vi "HMI CSE1.vi"() -> ()   [LabVIEW 2010]
uses:
  <vilib>/addons/Simulation Interface/_sitctls/sit Indicator Info.ctl
  <vilib>/addons/Simulation Interface/_sitctls/sit Indicator Type.ctl
  <vilib>/addons/Simulation Interface/_sitctls/sit Client Meta Info (v3).ctl
  <vilib>/addons/Simulation Interface/_sitctls/sit MDL Line Item Info.ctl
  <vilib>/addons/Simulation Interface/_sitctls/sit MDL Line Type.ctl
  <vilib>/addons/Simulation Interface/_sitctls/sit Details Settings.ctl
  <vilib>/addons/Simulation Interface/_sitctls/sit Execution Host.ctl
  <vilib>/addons/Simulation Interface/_sitctls/SIT Sim State.ctl
  <vilib>/Utility/inputDevices.llb/closeJoystick.vi
  <vilib>/Utility/inputDevices.llb/joystickAcquire.vi
  <vilib>/addons/Simulation Interface/_sitclient.llb/NI_SIT_sitclient.lvlib
  <vilib>/addons/Simulation Interface/_sitctls/NI_SIT_sitctls.lvlib
  <vilib>/ptbypt/NI_PtbyPt.lvlib
  <vilib>/picture/3D Picture Control/NI_3D Picture Control.lvlib
panel:
  out "Navigation eta yaw":dbl
  out "Navigation eta sway":dbl
  out "Navigation eta surge":dbl
  out "Plant u5":dbl
  out "Plant u4":dbl
  out "Plant u3":dbl
  out "Plant u2":dbl
  out "Plant u1":dbl
  out "DP eta Psi deg":dbl
  out "DP eta E":dbl
  out "DP eta N":dbl
  out "DP eta_d Psi deg":dbl
  out "DP eta_d E":dbl
  out "DP eta_d N":dbl
  in  "Enabler":bool
  in  "Enable Linear Simulator":bool
  in  "Control Input Selector":enum32{"OK Button 4", "OK Button 5"}(radio)
  in  "MODE":T1(radio)=enum."OK Button 4"
  in  "Enable CSE1 actuator":bool
  in  "SIT_RVE":bool
  in  "SIT_Remap":bool
  in  "SIT_Details":bool
  in  "SIT_Stop":bool
  in  "SIT_Pause":bool
  in  "SIT_Run":bool
  in  "SIT_stopVI":bool
  out "SIT_Status":string
  in  "Tab Front Pannel":T2(tab)
  in  "u5":dbl
  in  "u4":dbl
  in  "u3":dbl
  in  "u2":dbl
  in  "u1":dbl
  in  "VSP Speed":dbl(slide) min=-1.0 max=1.0 step=0.05 scale=-1.0..1.0 scale format="%#_2g"
  in  "BT Power Limiter":dbl(slide) min=0.0 max=1.0 step=0.1 scale=-1.0..1.0
  in  "Left Y":dbl(slide) scale=-35860.0..35860.0
  in  "Left X":dbl(slide) scale=-35860.0..35860.0
  in  "Right X":dbl(slide) scale=-35860.0..35860.0
  in  "Right Y":dbl(slide) scale=-35860.0..35860.0
  out "Servo Battery":dbl(knob) scale=0.0..8.0
  out "Bowthruster Battery":dbl(knob) scale=0.0..8.0
  out "Main Battery":dbl(knob) scale=0.0..18.0
  out "Left Joystick":bool
  out "Right Joystick":bool
  out "Direction Up":bool
  out "Direction Right":bool
  out "Direction Down":bool
  out "Direction Left":bool
  out "L2 Button":bool
  out "R2 Button":bool
  out "Triangle Button":bool
  out "Circle Button":bool
  out "X Button":bool
  out "Square Button":bool
  out "Joystick Info":T3(array[cluster])
  in  "L2":sgl
  in  "R2":sgl
  out "Slide BT red":dbl(slide)
  out "Slide BT green":dbl(slide) scale=0.0..1.0
  out "Magnitude Pitch Starboard VSP":dbl(knob) scale=0.0..1.0
  out "Magnitude Pitch Port VSP":dbl(knob) scale=0.0..1.0
  out "Direction Starboard VSP":dbl(knob) scale=180.0..-180.0
  out "Direction Port VSP":dbl(knob) scale=180.0..-180.0
  in  "Acccuracy BT":dbl
  in  "Accuracy VSP":dbl
  in  "Tab Plants":enum32{"eta", "Qualisys", "Linear Simulator"}(tab)
  in  "Tab eta":enum32{"Navigation output", "Qualisys"}(tab)
  out "Iceberg yaw":dbl
  out "Iceberg pitch":dbl
  out "Iceberg roll":dbl
  out "Iceberg z-position":dbl
  out "Iceberg y-position":dbl
  out "Iceberg x-position":dbl
  out "CSE1 yaw [rad]":dbl
  out "CSE1 pitch [rad]":dbl
  out "CSE1 roll [rad]":dbl
  out "CSE1 z-position [m]":dbl
  out "CSE1 y-position [m]":dbl
  out "CSE1 x-position [m]":dbl
  out "QS yaw [rad]":dbl
  out "QS pitch [rad]":dbl
  out "QS roll [rad]":dbl
  out "QS z-position [m]":dbl
  out "QS y-position [m]":dbl
  out "QS x-position [m]":dbl
  in  "Show CSEI":bool
  in  "Show Iceberg":bool
  out "QTM In9":dbl
  out "QTM In8":dbl
  out "QTM In7":dbl
  out "QTM In6":dbl
  out "QTM In5":dbl
  out "QTM In4":dbl
  out "QTM In3":dbl
  out "QTM In2":dbl
  out "QTM In1":dbl
  out "LS nu_yaw_hil":dbl
  out "LS nu_sway_hil":dbl
  out "LS nu_surge_hil":dbl
  out "LS etadot_yaw_hil":dbl
  out "LS etadot_sway_hil":dbl
  out "LS etadot_surge_hil":dbl
  out "LS eta_yaw_hil":dbl
  out "LS eta_sway_hil":dbl
  out "LS  eta_surge_hil":dbl
  in  "LS r_0":dbl
  in  "LS v_0":dbl
  in  "LS u_0":dbl
  in  "LS psi_0":dbl
  in  "LS y_0":dbl
  in  "LS x_0":dbl
  in  "Button Reset HIL Integrator":bool
  in  "Reset Linear Simulator integrator":dbl
  in  "Tab Control system":enum32{"DP Control", "Page 2"}(tab)
  in  "DP Wave Filter":bool
  in  "DP eta_d LPF":bool
  in  "DP K_d Scale":dbl(slide) min=0.0 max=5.0 step=0.25 scale=0.0..5.0
  in  "DP K_i Scale":dbl(slide) min=0.0 max=5.0 step=0.25 scale=0.0..5.0
  in  "DP K_p Scale":dbl(slide) min=0.0 max=10.0 step=0.5 scale=0.0..10.0
  in  "DP eta_d_N [m]":dbl
  in  "DP eta_d_E [m]":dbl
  in  "Button Reset DP Integrator.":bool
  in  "DP eta_d_Psi [deg]":dbl(knob) scale=0.0..360.0 scale format="%#.3p"
  out "Ind eta_d_Psi [rad]":dbl format="%#_2g"
  in  "Reset DP Integrator":dbl
  out "3D Picture":refnum<vi>(3d-picture)
  in  "Tab Reg plots":enum32{"DP", "Page 2"}(tab)
  out "DP Reponse N":cluster{"Value":dbl, "Value":dbl}(graph)
  out "DP Error N":waveform(dbl)[](graph)
  out "DP Error E":waveform(dbl)[](graph)
  out "DP Error Psi":waveform(dbl)[](graph)
  out "DP Reponse Psi":cluster{"Value":dbl, "Value":dbl}(graph)
  out "DP Response E":cluster{"Value":dbl, "Value":dbl}(graph)
  in  "Tab Command":enum32{"DP", "Page 2"}(tab)
  out "DP tau surge":waveform(dbl)[](graph)
  out "DP tau sway":waveform(dbl)[](graph)
  out "DP tau yaw":waveform(dbl)[](graph)
  out "DP u_1":waveform(dbl)[](graph)
  out "DP u_2":waveform(dbl)[](graph)
  out "DP u_3":waveform(dbl)[](graph)
  out "DP u_4":waveform(dbl)[](graph)
  out "DP u_5":waveform(dbl)[](graph)
  in  "SIT_Meta_Info":T4
  in  "SIT_Indicator_Indices":T9[](array[typedef])=[{"Indicator Index"=0, "Number of Signals"=1, "Indicator Type"=enum."Knob"}, {"Indicator Index"=-1, "Number of Signals"=0, "Indicator Type"=enum."Digital"}, {"Indicator Index"=-1, "Number of Signals"=0, "Indicator Type"=enum."Digital"}, {"Indicator Index"=3, "Number of Signals"=1, "Indicator Type"=enum."Digital"}, {"Indicator Index"=4, "Number of Signals"=1, "Indicator Type"=enum."Digital"}, {"Indicator Index"=5, "Number of Signals"=1, "Indicator Type"=enum."Digital"}, {"Indicator Index"=-1, "Number of Signals"=0, "Indicator Type"=enum."Digital"}, {"Indicator Index"=7, "Number of Signals"=1, "Indicator Type"=enum."WaveformChart"}, {"Indicator Index"=8, "Number of Signals"=1, "Indicator Type"=enum."WaveformChart"}, {"Indicator Index"=9, "Number of Signals"=1, "Indicator Type"=enum."WaveformChart"}, {"Indicator Index"=10, "Number of Signals"=1, "Indicator Type"=enum."Digital"}, {"Indicator Index"=11, "Number of Signals"=1, "Indicator Type"=enum."Digital"}, {"Indicator Index"=12, "Number of Signals"=1, "Indicator Type"=enum."Digital"}, {"Indicator Index"=13, "Number of Signals"=1, "Indicator Type"=enum."Digital"}, {"Indicator Index"=14, "Number of Signals"=1, "Indicator Type"=enum."Digital"}, {"Indicator Index"=15, "Number of Signals"=1, "Indicator Type"=enum."Digital"}, {"Indicator Index"=16, "Number of Signals"=1, "Indicator Type"=enum."WaveformChart"}, {"Indicator Index"=17, "Number of Signals"=1, "Indicator Type"=enum."WaveformChart"}, {"Indicator Index"=18, "Number of Signals"=1, "Indicator Type"=enum."WaveformChart"}, {"Indicator Index"=19, "Number of Signals"=1, "Indicator Type"=enum."WaveformChart"}, {"Indicator Index"=20, "Number of Signals"=1, "Indicator Type"=enum."WaveformChart"}, {"Indicator Index"=21, "Number of Signals"=1, "Indicator Type"=enum."WaveformChart"}, {"Indicator Index"=22, "Number of Signals"=1, "Indicator Type"=enum."WaveformChart"}, {"Indicator Index"=23, "Number of Signals"=1, "Indicator Type"=enum."WaveformChart"}, {"Indicator Index"=24, "Number of Signals"=1, "Indicator Type"=enum."Knob"}, {"Indicator Index"=25, "Number of Signals"=1, "Indicator Type"=enum."Knob"}, {"Indicator Index"=-1, "Number of Signals"=0, "Indicator Type"=enum."Digital"}, {"Indicator Index"=-1, "Number of Signals"=0, "Indicator Type"=enum."Digital"}, {"Indicator Index"=-1, "Number of Signals"=0, "Indicator Type"=enum."Digital"}, {"Indicator Index"=-1, "Number of Signals"=0, "Indicator Type"=enum."Digital"}, {"Indicator Index"=-1, "Number of Signals"=0, "Indicator Type"=enum."Digital"}, {"Indicator Index"=-1, "Number of Signals"=0, "Indicator Type"=enum."Digital"}, {"Indicator Index"=32, "Number of Signals"=1, "Indicator Type"=enum."Digital"}, {"Indicator Index"=33, "Number of Signals"=1, "Indicator Type"=enum."Digital"}, {"Indicator Index"=34, "Number of Signals"=1, "Indicator Type"=enum."Digital"}, {"Indicator Index"=35, "Number of Signals"=1, "Indicator Type"=enum."Digital"}, {"Indicator Index"=36, "Number of Signals"=1, "Indicator Type"=enum."Digital"}, {"Indicator Index"=37, "Number of Signals"=1, "Indicator Type"=enum."Digital"}, {"Indicator Index"=38, "Number of Signals"=1, "Indicator Type"=enum."Digital"}, {"Indicator Index"=39, "Number of Signals"=1, "Indicator Type"=enum."Digital"}, {"Indicator Index"=40, "Number of Signals"=1, "Indicator Type"=enum."Digital"}, {"Indicator Index"=41, "Number of Signals"=1, "Indicator Type"=enum."Knob"}, {"Indicator Index"=42, "Number of Signals"=1, "Indicator Type"=enum."Knob"}, {"Indicator Index"=43, "Number of Signals"=1, "Indicator Type"=enum."Knob"}, {"Indicator Index"=44, "Number of Signals"=1, "Indicator Type"=enum."Digital"}, {"Indicator Index"=45, "Number of Signals"=1, "Indicator Type"=enum."Digital"}, {"Indicator Index"=46, "Number of Signals"=1, "Indicator Type"=enum."Digital"}, {"Indicator Index"=47, "Number of Signals"=1, "Indicator Type"=enum."Digital"}, {"Indicator Index"=48, "Number of Signals"=1, "Indicator Type"=enum."Digital"}, {"Indicator Index"=49, "Number of Signals"=1, "Indicator Type"=enum."Digital"}, {"Indicator Index"=50, "Number of Signals"=1, "Indicator Type"=enum."Digital"}, {"Indicator Index"=51, "Number of Signals"=1, "Indicator Type"=enum."Digital"}, {"Indicator Index"=52, "Number of Signals"=1, "Indicator Type"=enum."Digital"}, {"Indicator Index"=53, "Number of Signals"=1, "Indicator Type"=enum."Digital"}, {"Indicator Index"=54, "Number of Signals"=1, "Indicator Type"=enum."Digital"}, {"Indicator Index"=55, "Number of Signals"=1, "Indicator Type"=enum."Digital"}, {"Indicator Index"=56, "Number of Signals"=1, "Indicator Type"=enum."Digital"}, {"Indicator Index"=57, "Number of Signals"=1, "Indicator Type"=enum."Digital"}, {"Indicator Index"=58, "Number of Signals"=1, "Indicator Type"=enum."Digital"}, {"Indicator Index"=59, "Number of Signals"=1, "Indicator Type"=enum."Digital"}, {"Indicator Index"=60, "Number of Signals"=1, "Indicator Type"=enum."Digital"}, {"Indicator Index"=61, "Number of Signals"=1, "Indicator Type"=enum."Digital"}, {"Indicator Index"=62, "Number of Signals"=1, "Indicator Type"=enum."Digital"}, {"Indicator Index"=63, "Number of Signals"=1, "Indicator Type"=enum."Digital"}, {"Indicator Index"=64, "Number of Signals"=1, "Indicator Type"=enum."Digital"}, {"Indicator Index"=65, "Number of Signals"=1, "Indicator Type"=enum."Digital"}, {"Indicator Index"=66, "Number of Signals"=1, "Indicator Type"=enum."Digital"}, {"Indicator Index"=67, "Number of Signals"=1, "Indicator Type"=enum."Knob"}, {"Indicator Index"=68, "Number of Signals"=1, "Indicator Type"=enum."Slide"}, {"Indicator Index"=69, "Number of Signals"=1, "Indicator Type"=enum."Slide"}]
  # "MODE"
  # "Controller Input Selector"
  # "TARGET"
  # "Model Controls"
  # "VSP Speed"
  # "VSP speed = 1\n\nStarboard VSP\nMax Speed  ClockWise\n\nPort VSP \nMax Speed CounterClockWise"
  # "VSP Speed = -1\n\nStarboard VSP \nMax Speed CounterClockWise\n\nPort VSP\nMax Speed ClockWise"
  # "Bow Thruster Power Limit"
  # "Max Power"
  # "Max Power"
  # "No Power"
  # "PS3 Joysticks"
  # "Increase BT power limit"
  # "Increase VSP speed"
  # "Decrease BT power limit"
  # "Decrease VSP speed"
  # "Port VSP\n(surge/sway force setpoint)"
  # "Starboard VSP"
  # "Bowthruster"
  # "VSP pitch"
  # "CS Enterprise I"
  # "Toggle visibility"
  # "Iceberg"
  # "Toggle visibility"
  # "Initial eta"
  # "Initial nu"
  # "DP controller gains"
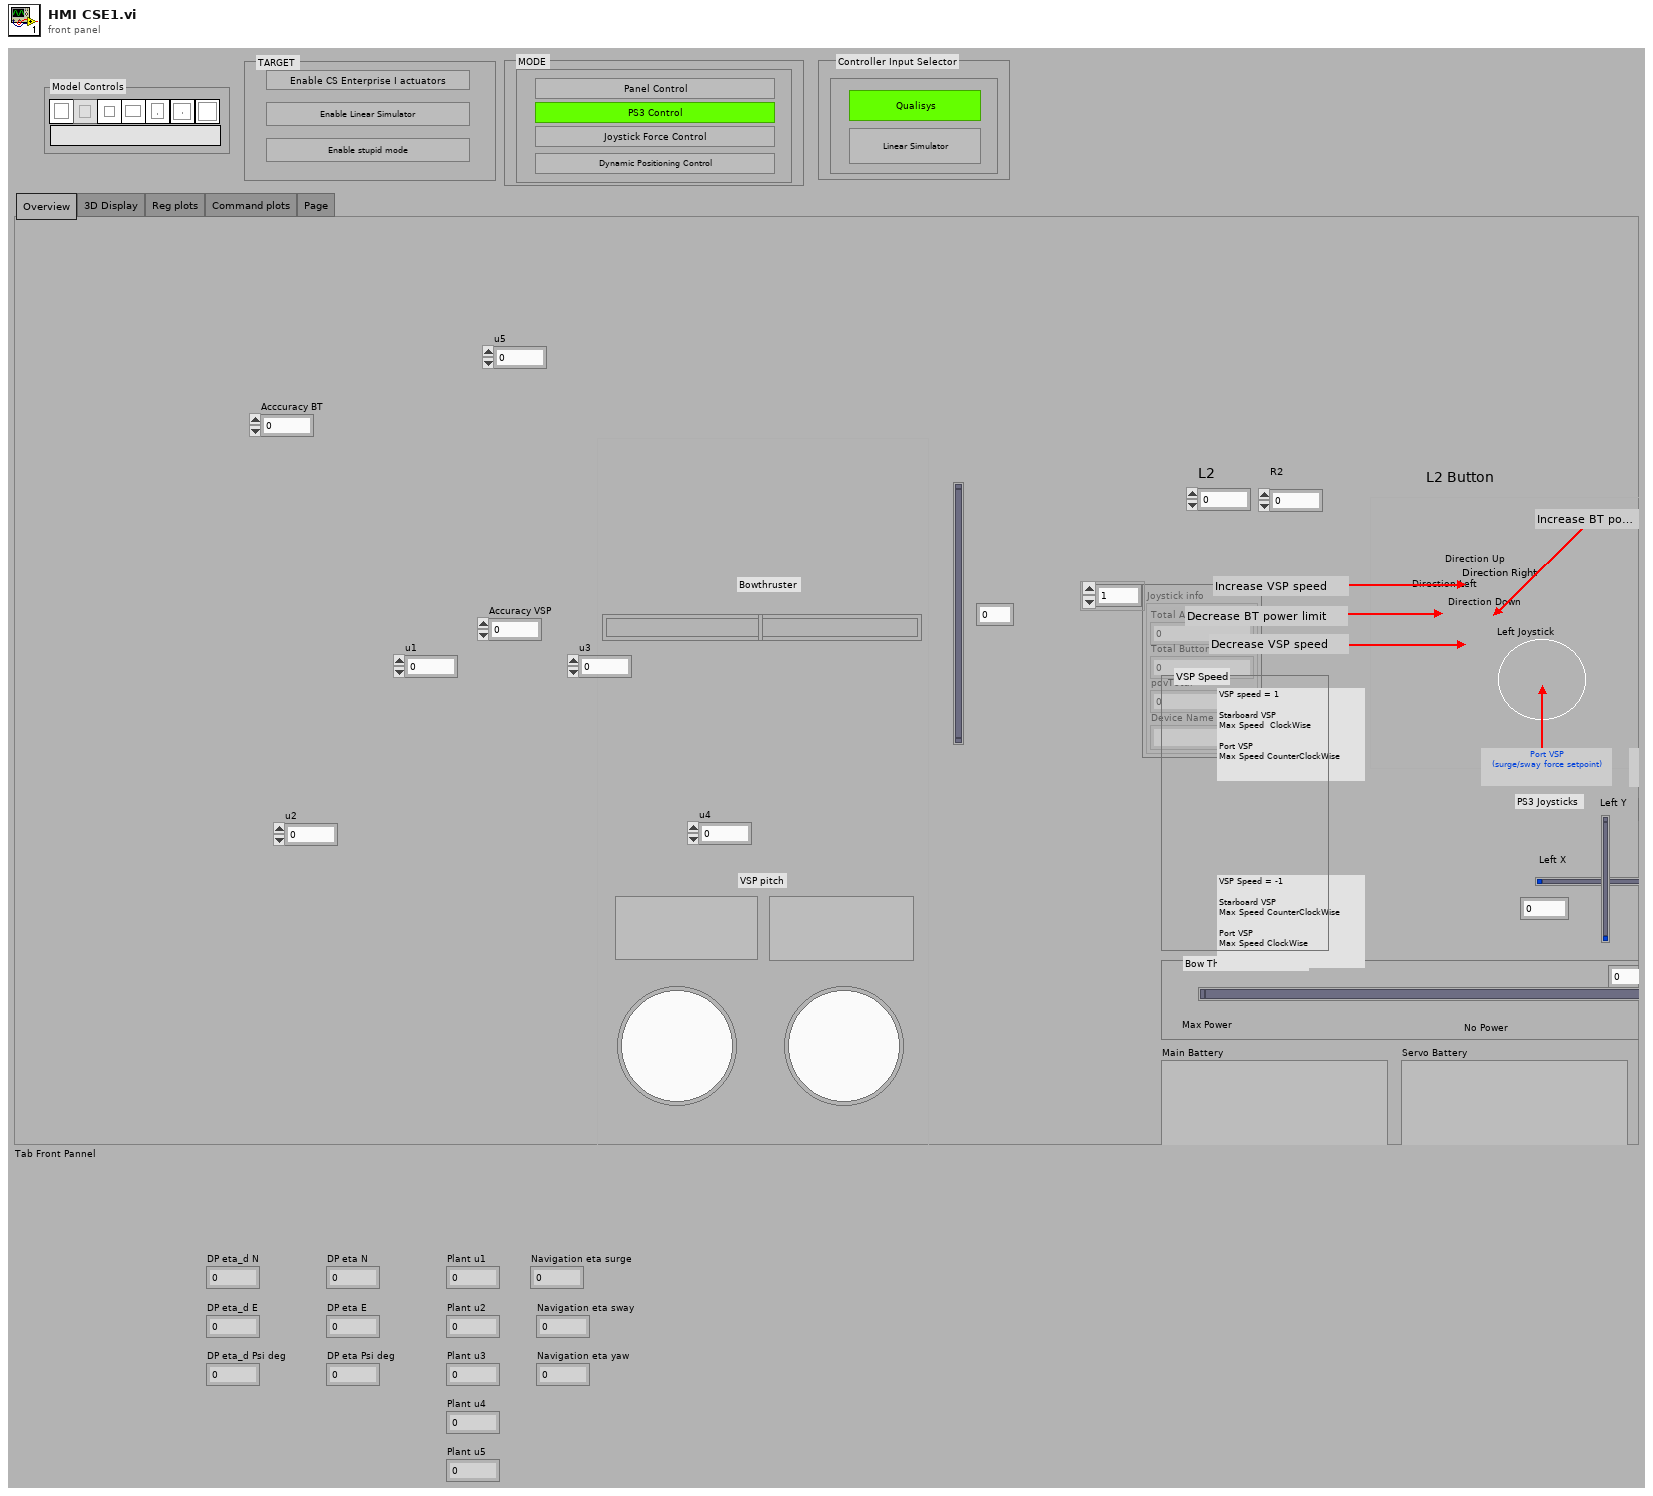
[diagram p1: front panel]
types:
  T1 = enum32{"Radio Selection 4", "OK Button 4", "OK Button 5", "OK Button 6"}
  T2 = enum32{"Overview", "3D Display", "Reg plots", "Command plots", "Page"}
  T3 = cluster{"Total Axis":u32, "Total Buttons":u32, "povTotal":u32, "Device Name":string}[]
  T4 = typedef "NI_SIT_sitctls.lvlib/sit Client Meta Info (v3).ctl" = cluster{"Simulation IP":string, "Target IP":string, "Host Port":u16, "Model DLL Path":path, "Model File Path":path, "Model Name":string, "Param Tree Info ":T5[], "Signal Tree Info":T5[], "Details Settings":T7, "Client Name":string, "Stored Model Checksum":string, "Buffer Sizes":cluster{"number of signals":u32, "circular buffer size":u32, "num data points":u32}, "Execution Host":T8, "Project Dir":path, "Last MDL":path}
  T5 = typedef "NI_SIT_sitctls.lvlib/sit MDL Line Item Info.ctl" = cluster{"Line Type":T6, "Section Type":string, "Name":string, "Value":string, "Owner Index":i32, "Tree Tag":string, "Child Indices":i32[], "Expanded?":bool, "Destination Block Info":string[]}
  T6 = typedef "NI_SIT_sitctls.lvlib/sit MDL Line Type.ctl" = enum16{"Section Head", "Parameter", "Section End", "Comment"}
  T7 = typedef "NI_SIT_sitctls.lvlib/sit Details Settings.ctl" = cluster{"Halt on Task Overrun?":bool, "Halt on Lost Data?":bool, "Signal Decimation":i32, "Autoscale":bool}
  T8 = typedef "NI_SIT_sitctls.lvlib/sit Execution Host.ctl" = enum32{"Simulation Environment", "RT Target", "Local Driver"}
  T9 = typedef "NI_SIT_sitctls.lvlib/sit Indicator Info.ctl" = cluster{"Indicator Index":i32, "Number of Signals":i32, "Indicator Type":T10}
  T10 = typedef "NI_SIT_sitctls.lvlib/sit Indicator Type.ctl" = enum32{"xxx1", "xxx2", "xxx3", "Generic   ", "Decoration", "Text", "xControl", "ColorBox", "Boolean", "RefNum", "Variant", "Path", "ListBox", "Table", "Array", "Picture", "ActiveXContainer", "Numeric", "Digital", "NamedNumeric", "ColorRamp", "Slide", "GraphOrChart", "WaveformChart", "WaveformGraph", "IntensityChart", "xxx4", "xxx5", "xxx6", "xxx7", "Cluster", "Panel", "Knob", "NumWithScale", "Ring", "Enum", "GObject", "Plot", "Cursor", "NumericText", "Scale", "ColorScale", "GraphScale", "ColorGraphScale", "TypedRefNum", "OldKnobScale", "MCListbox", "WaveformData", "BVTag", "DAQName", "VISAName", "IVIName", "SlideScale"}
  T11 = cluster{"Red":sgl, "Green":sgl, "Blue":sgl, "Alpha":sgl}
  T12 = cluster{"axes total":u32, "buttons total":u32, "pov total":u32, "device name":string}[]
  T13 = typedef "NI_SIT_sitctls.lvlib/sit TCP Conn and Queue.ctl" = cluster{"TCP Connection":refnum<k5>, "Data Queue":refnum<queue>, "Execution Host":T8}
  T14 = typedef "NI_SIT_sitctls.lvlib/sit Client Op Refs.ctl" = cluster{"Conn and Queue":T13, "RunPauseStop Refs":refnum<vi>[], "Control Refs":refnum<vi>[], "Indicator Refs":refnum<vi>[], "Param Info":T15[], "State Queue":refnum<queue>, "Don't Modify Scales?":bool, "Param Info Needs Init?":bool}
  T15 = typedef "NI_SIT_sitctls.lvlib/SIT param info.ctl" = cluster{"paramidx":i32, "ID":string, "paramname":string, "dattype":i32, "Dimensions":i32[], "value":dbl[]}
  T16 = typedef "NI_SIT_sitctls.lvlib/SIT Sim State.ctl" = enum8{"Default", "Idle", "Running", "Paused", "Stopped", "Error"}
  T17 = cluster{"X axis":i32, "Y axis":i32, "Z axis":i32, "X axis rotation":i32, "Y axis rotation":i32, "Z axis rotation":i32, "U axis":i32, "V axis":i32}
  T18 = cluster{"button 1":bool, "button 2":bool, "button 3":bool, "button 4":bool, "button 5":bool, "button 6":bool, "button 7":bool, "button 8":bool, "button 9":bool, "button 10":bool, "button 11":bool, "button 12":bool, "button 13":bool, "button 14":bool, "button 15":bool, "button 16":bool, "button 17":bool, "button 18":bool, "button 19":bool, "button 20":bool, "button 21":bool, "button 22":bool, "button 23":bool, "button 24":bool, "button 25":bool, "button 26":bool, "button 27":bool, "button 28":bool, "button 29":bool, "button 30":bool, "button 31":bool, "button 32":bool}
  T19 = cluster{"pov 1":i32, "pov 2":i32, "pov 3":i32, "pov 4":i32}
  T20 = cluster{"DP eta_d_N [m]":dbl, "Red":sgl, "DP eta_d_E [m]":dbl}
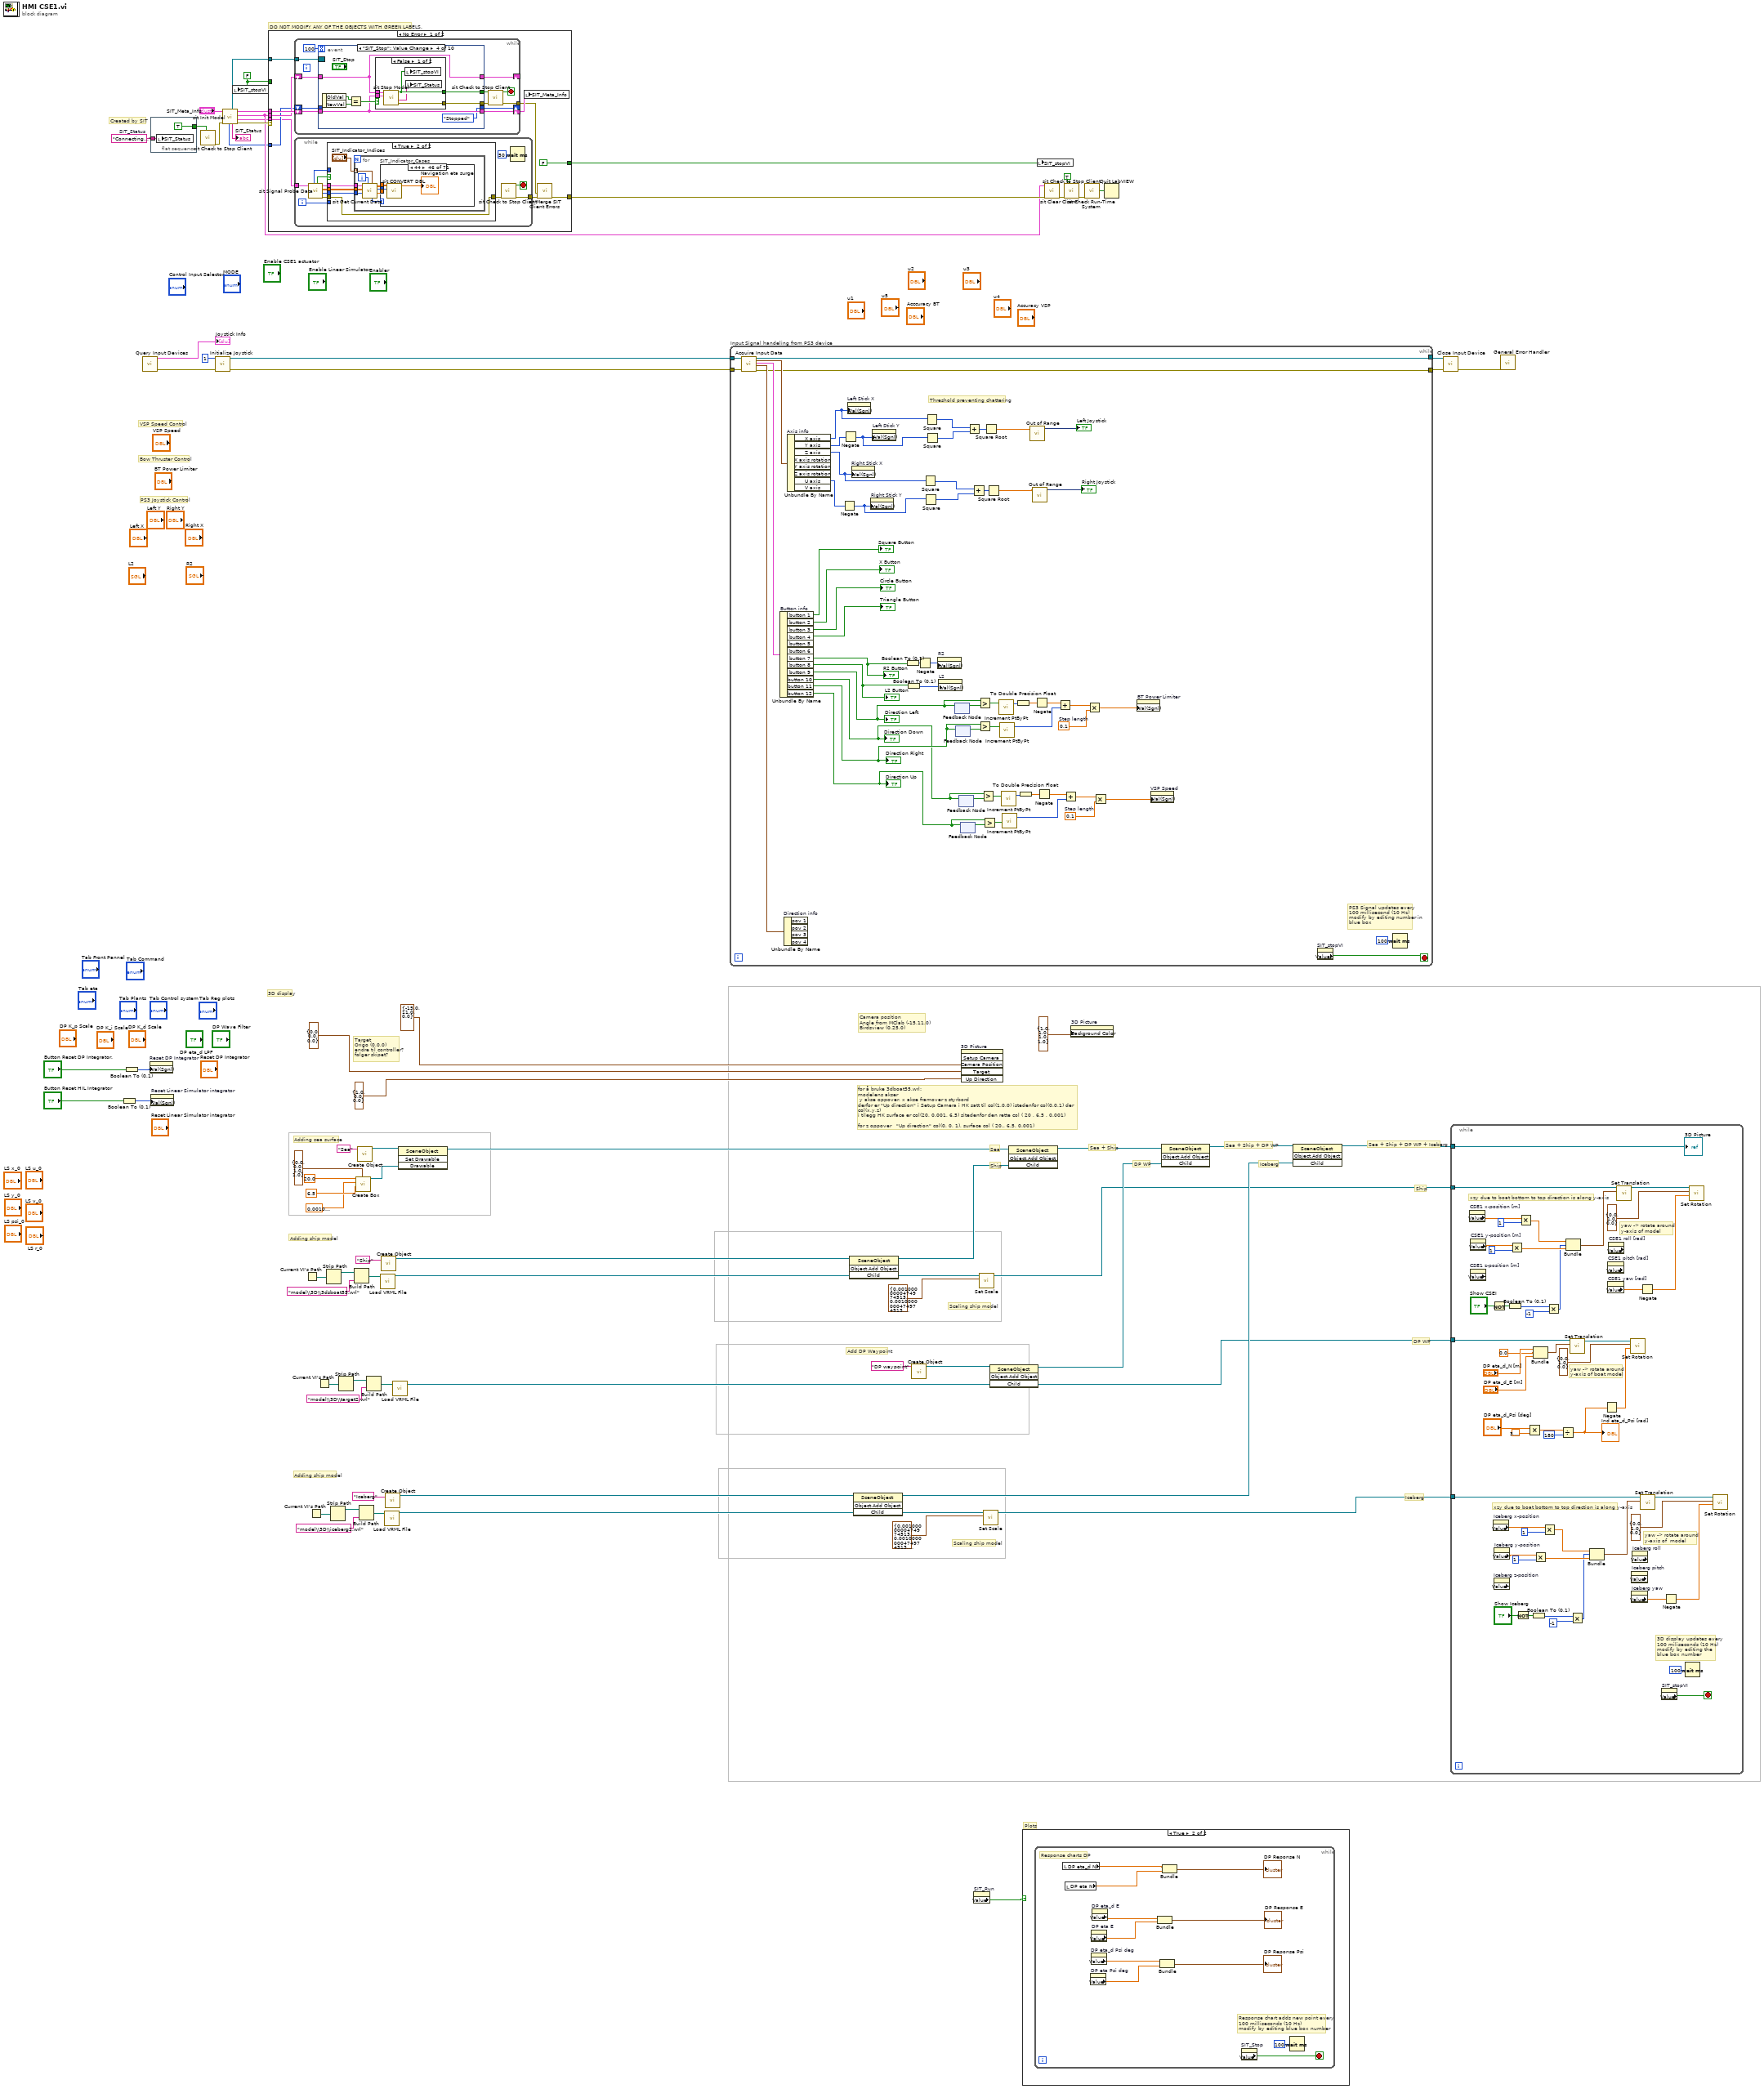
[diagram p0: block diagram]
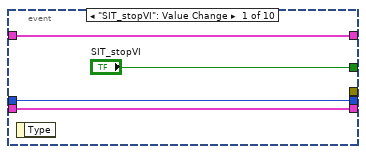
[diagram p3: hidden frame]
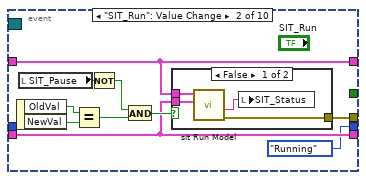
[diagram p4: hidden frame]
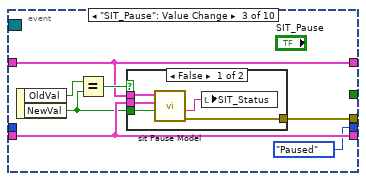
[diagram p6: hidden frame]
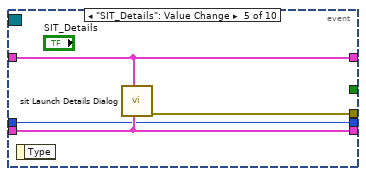
[diagram p9: hidden frame]
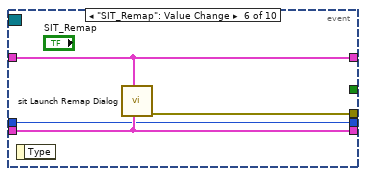
[diagram p10: hidden frame]
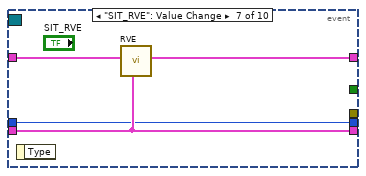
[diagram p11: hidden frame]
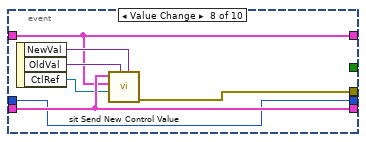
[diagram p12: hidden frame]
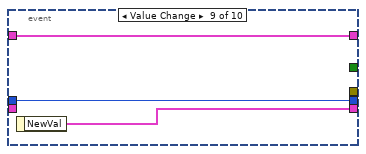
[diagram p13: hidden frame]
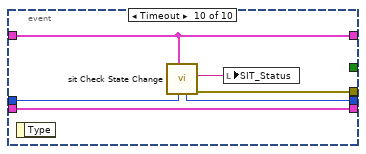
[diagram p14: hidden frame]
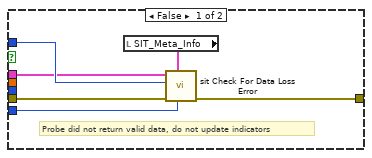
[diagram p15: hidden frame]
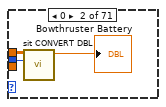
[diagram p17: hidden frame]
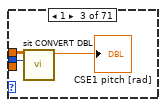
[diagram p18: hidden frame]
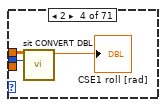
[diagram p19: hidden frame]
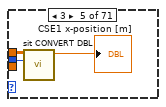
[diagram p20: hidden frame]
diagram:
  w62 = "Connecting..."  # SIT_Status
  w67 = FALSE
  # "Plots"
  # "Iceberg"
  # "Iceberg"
  # "Sea + Ship + DP WP + Iceberg"
  # "Scaling ship model"
  # "Adding ship model"
  # "DP WP"
  # "Ship"
  # "3D display"
  # "DP WP"
  # "Target\nOrigo (0,0,0)\nendre til controller?\nfølger skipet?"
  # "Scaling ship model"
  # "Camera position\nAngle from MClab (-15,11,0)\nBirdsview (0,25,0)"
  # "Add DP Waypoint"
  # "Sea + Ship + DP WP"
  # "for å bruke 3dboat55.wrl:\nmodelens akser\n y akse oppover, x akse framover z styrbord\nderfor er \"Up direction\" i Setup Camera i HK satt til col(1,0,0) istedenfor col(0,0,1) der col(x,y,z)\ni tilegg HK surface er col(20, 0.001, 6.5) sitedenfor den rette col ( 20 , 6.5 , 0.001) \n\nfor z oppover   \"Up direction\" col(0, 0, 1), surface col ( 20., 6.5, 0.001)"
  # "Sea + Ship"
  # "Ship"
  # "Sea"
  # "Adding sea surface"
  # "Adding ship model"
  # "VSP Speed Control"
  # "Bow Thruster Control"
  # "Created by SIT"
  # "PS3 Joystick Control"
  # "DO NOT MODIFY ANY OF THE OBJECTS WITH GREEN LABELS."
  n1 = Boolean To (0,1)(Boolean="Button Reset HIL Integrator") -> (0, 1=w4:i16)
  n2 = Boolean To (0,1)(Boolean="Button Reset DP Integrator.") -> (0, 1=w2:i16)
  n3 = call <vilib>:"Query Input Devices.vi"() -> ("error out"=w56:errorcluster, "joystick info"=→"Joystick Info":T12)  [unwired: 8 in, 2 out]
  n4 = property on="Reset DP Integrator" class="DigNum (strict)"("Val(Sgnl)"=w2) -> ()  [unwired: 2 in, 2 out]
  n5 = flat-sequence {
    tunnel: [TRUE ("Clear Item?")] -> w71
    tunnel: w62 -> [w78]
    frame #0 {
      n6 = local write "SIT_Status"(w78) -> ()
    }
  }
  n7 = property on="Reset Linear Simulator integrator" class="DigNum (strict)"("Val(Sgnl)"=w4) -> ()  [unwired: 2 in, 2 out]
  n8 = call <vilib>:"sit Check to Stop Client.vi"("Reset Stop?"=w71) -> ("error out"=w73:errorcluster)  [unwired: 2 in, 8 out]
  n9 = call <vilib>:"Initialize Joystick.vi"("error in (no error)"=w56, "device index"=1) -> ("error out"=w58:errorcluster, "device ID"=w59:refnum<k1>)  [unwired: 8 in]
  n10 = call <vilib>:"sit Init Model.vi"("error in (no error)"=w73, "SIT_Meta_Info in"="SIT_Meta_Info") -> ("error out"=w77:errorcluster, "Conn and Queue"=w64:T13, "SIT Client Op Refs"=w68:T14, "SIT_Meta_Info out"=w75:T4, "Initial State"=→"SIT_Status":string, "Event Registration Refnum"=w76:refnum<event-registration>, "State"=w65:T16)  [unwired: 2 in, 1 out]
  n11 = local write "SIT_stopVI"(w67) -> ()
  n12 = case shown="No Error" w77 {
    selector: w77 -> [_ w438]
    tunnel: w76 -> [w89 _]
    tunnel: w75 -> [w87 w437]
    tunnel: [w83 w438] -> w72
    tunnel: w68 -> [w86 _]
    tunnel: w67 -> [_ _]
    tunnel: [FALSE _] -> w66
    tunnel: w65 -> [w81 _]
    tunnel: w64 -> [w80 _]
    frame No Error {
      n13 = while {
        tunnel: w89 -> [w101]
        tunnel: [w99] -> w82
        shift-right: [w93] -> _
        shift-left: w86 -> [w97]
        shift-right: [w100] -> w88
        shift-left: w87 -> [w98]
        shift-right: [w90] -> _
        shift-left: w81 -> [w91]
        stop <- w92 stop-if-true
        n14 = event shown="[3] \"SIT_Stop\": Value Change" {
          selector: w101 -> [_ _ _ _ _ _ _ _ _ _]
          dyn-events: _ -> [_ _ _ _ _ _ _ _ _ _]
          timeout: 100 -> [_ _ _ _ _ _ _ _ _ _]
          tunnel: ["SIT_stopVI" _ _ w136 _ _ _ _ _ _] -> w94
          tunnel: [_ w111 w123 w135 w148 w152 _ w163 _ w170] -> w95
          tunnel: w98 -> [w104 w109 w124 w137 w147 w151 w155 w162 _ w172]
          tunnel: w97 -> [w102 w110 w125 w138 w146 w149 w156 w158 w165 w171]
          tunnel: [w104 w109 w124 w137 w147 w151 w155 w162 w166 w172] -> w100
          tunnel: [w102 w110 w125 w138 w146 w149 w154 w158 w165 w171] -> w93
          tunnel: [w103 SIT_Sim_State."Running" ("State") SIT_Sim_State."Paused" ("State") SIT_Sim_State."Stopped" ("State") w145 w150 w153 w157 w164 w168] -> w90
          tunnel: w91 -> [w103 _ _ _ w145 w150 w153 w157 w164 w169]
          event "SIT_stopVI": Value Change {
            n15 = event-data() -> ()  [unwired: 2 out]
          }
          event "SIT_Run": Value Change {
            n16 = event-data() -> ("OldVal"=w107:bool, "NewVal"=w108:bool)  [unwired: 1 out]
            n17 = local read "SIT_Pause"() -> (w114:bool)
            n18 = Equal?(x=w107, y=w108) -> (x = y?=w112:bool)
            n19 = Not(x=w114) -> (.not. x?=w115:bool)
            n20 = And(x=w115, y=w112) -> (x .and. y?=w113:bool)
            n21 = case shown="False" w113 {
              tunnel: [w119 _] -> w111
              tunnel: w110 -> [w118 _]
              tunnel: w109 -> [w117 _]
              frame False {
                n22 = call <vilib>:"sit Run Model.vi"("SIT Meta Info"=w117, "SIT Client Op Refs"=w118) -> ("error out"=w119:errorcluster, "Status"=w116:string)  [unwired: 6 in, 2 out]
                n23 = local write "SIT_Status"(w116) -> ()
              }
              frame True {
                # "Ignore value change if it is\nto the same value"
              }
            }
          }
          event "SIT_Pause": Value Change {
            n24 = event-data() -> ("OldVal"=w121:bool, "NewVal"=w122:bool)  [unwired: 1 out]
            n25 = Equal?(x=w121, y=w122) -> (x = y?=w126:bool)
            n26 = case shown="False" w126 {
              tunnel: [w131 _] -> w123
              tunnel: w125 -> [w130 _]
              tunnel: w124 -> [w129 _]
              tunnel: w122 -> [w128 _]
              frame False {
                n27 = call <vilib>:"sit Pause Model.vi"("Pause Button Value"=w128, "SIT Meta Info"=w129, "SIT Client Op Refs"=w130) -> ("error out"=w131:errorcluster, "Status"=w127:string)  [unwired: 3 in, 4 out]
                n28 = local write "SIT_Status"(w127) -> ()
              }
              frame True {
                # "Ignore value change if it is\nto the same value"
              }
            }
          }
          event "SIT_Stop": Value Change {
            n29 = event-data() -> ("OldVal"=w133:bool, "NewVal"=w134:bool)  [unwired: 1 out]
            n30 = Equal?(x=w133, y=w134) -> (x = y?=w139:bool)
            n31 = case shown="False" w139 {
              tunnel: [w144 _] -> w135
              tunnel: [w141 _] -> w136
              tunnel: w137 -> [w143 _]
              tunnel: w138 -> [w142 _]
              frame False {
                n32 = call <vilib>:"sit Stop Model.vi"("SIT Meta Info"=w143, "SIT Client Op Refs"=w142) -> ("error out"=w144:errorcluster, "Status"=w140:string, "Stop VI?"=w141:bool)  [unwired: 4 in, 3 out]
                n33 = local write "SIT_stopVI"(w141) -> ()
                n34 = local write "SIT_Status"(w140) -> ()
              }
              frame True {
                # "Ignore value change if it is\nto the same value"
              }
            }
          }
          event "SIT_Details": Value Change {
            n35 = event-data() -> ()  [unwired: 2 out]
            n36 = call <vilib>:"sit Launch Details Dialog.vi"("SIT Meta Info in"=w147, "SIT Client Op Refs"=w146) -> ("error out"=w148:errorcluster)  [unwired: 1 in, 8 out]
          }
          event "SIT_Remap": Value Change {
            n37 = event-data() -> ()  [unwired: 2 out]
            n38 = call <vilib>:"sit Launch Remap Dialog.vi"("SIT Meta Info in"=w151, "SIT Client Op Refs"=w149) -> ("error out"=w152:errorcluster)  [unwired: 2 in, 7 out]
          }
          event "SIT_RVE": Value Change {
            n39 = event-data() -> ()  [unwired: 2 out]
            n40 = call <vilib>:"RVE.vi"("SIT_Meta_Info"=w155, "SIT Client Op Refs in"=w156) -> ("SIT Client Op Refs out"=w154:T14)  [unwired: 9 out]
          }
          event Value Change {
            n41 = event-data() -> ("NewVal"=w159:variant, "OldVal"=w160:variant, "CtlRef"=w161:refnum<vi>)  [unwired: 1 out]
            n42 = call <vilib>:"sit Send New Control Value.vi"("Control New Value"=w159, "Control Old Value"=w160, "Control Ref"=w161, "SIT Client Op Refs"=w158, "SIT_Meta_Info"=w162) -> ("error out"=w163:errorcluster)  [unwired: 4 in, 2 out]
          }
          event Value Change {
            n43 = event-data() -> ("NewVal"=w166:T4)  [unwired: 1 out]
          }
          event Timeout {
            n44 = event-data() -> ()  [unwired: 2 out]
            n45 = call <vilib>:"sit Check State Change.vi"("Old State in"=w169, "SIT Client Op Refs"=w171) -> ("error out"=w170:errorcluster, "Status String"=w167:string, "New State out"=w168:T16)  [unwired: 7 out]
            n46 = local write "SIT_Status"(w167) -> ()
          }
        }
        n47 = call <vilib>:"sit Check to Stop Client.vi"("error in (no error)"=w95, "User Stop?"=w94) -> ("error out"=w99:errorcluster, "Stop?"=w92:bool)  [unwired: 1 in, 7 out]
      }
      n48 = while "Read Loop" {
        tunnel: [w183] -> w84
        tunnel: w80 -> [w173]
        i -> [w180]
        stop <- w181 stop-if-true
        n49 = call <vilib>:"sit Signal Probe Data.vi"("TCP Conn and Queue"=w173) -> ("error out"=w176:errorcluster, "Dimensions"=w177:i32[], "Raw Data"=w178:dbl[][], "dup TCP Conn and Queue"=w179:T13, "Valid Data?"=w174:bool, "Options out"=w175:u32)  [unwired: 4 in, 1 out]
        n50 = case shown="True" w174 {
          tunnel: w178 -> [_ w194]
          tunnel: w177 -> [_ w193]
          tunnel: w179 -> [w186 w192]
          tunnel: w176 -> [w189 w191]
          tunnel: [w188 w191] -> w182
          tunnel: w175 -> [w190 _]
          tunnel: w180 -> [w187 _]
          frame False {
            # "Probe did not return valid data, do not update indicators"
            n51 = local read "SIT_Meta_Info"() -> (w185:T4)
            n52 = call <vilib>:"sit Check For Data Loss Error.vi"("Iteration"=w187, "SIT Meta Info"=w185, "error in (no error)"=w189, "Options"=w190, "TCP Conn and Queue"=w186) -> ("error out"=w188:errorcluster)  [unwired: 6 out]
          }
          frame True {
            n53 = for {
              tunnel: w194 -> [w204]
              tunnel: "SIT_Indicator_Indices" -> [w200] mode=indexing
              tunnel: w193 -> [w203]
              tunnel: w192 -> [w201]
              i -> [w202]
              n54 = call <vilib>:"sit Get Current Data.vi"("Indicator Index Cluster"=w200, "Iteration"=w202, "Dimensions"=w203, "Raw Data"=w204, "Conn and Queue"=w201) -> ("Timestamps"=w197:dbl[], "Last Row"=w198:i32, "Current Data"=w199:dbl[][], "Indicator Index"=w196:i32)  [unwired: 1 in, 2 out]
              n55 = case "SIT_Indicator_Cases" shown="44" w196 {
                tunnel: w199 -> [_ w207 w210 w213 w216 w219 w222 w225 w229 w234 w239 w243 w246 w249 w252 w255 w258 w262 w267 w272 w277 w282 w287 w292 w297 w301 w304 w307 w310 w313 w316 w319 w322 w325 w328 w331 w334 w337 w340 w343 w346 w349 w352 w355 w358 w361 w364 w367 w370 w373 w376 w379 w382 w385 w388 w391 w394 w397 w400 w403 w406 w409 w412 w415 w418 w421 w424 w427 w430 w433 w436]
                tunnel: w198 -> [_ w206 w209 w212 w215 w218 w221 w224 w228 w233 w238 w242 w245 w248 w251 w254 w257 w261 w266 w271 w276 w281 w286 w291 w296 w300 w303 w306 w309 w312 w315 w318 w321 w324 w327 w330 w333 w336 w339 w342 w345 w348 w351 w354 w357 w360 w363 w366 w369 w372 w375 w378 w381 w384 w387 w390 w393 w396 w399 w402 w405 w408 w411 w414 w417 w420 w423 w426 w429 w432 w435]
                tunnel: w197 -> [_ _ _ _ _ _ _ _ w227 w232 w237 _ _ _ _ _ _ w260 w265 w270 w275 w280 w285 w290 w295 _ _ _ _ _ _ _ _ _ _ _ _ _ _ _ _ _ _ _ _ _ _ _ _ _ _ _ _ _ _ _ _ _ _ _ _ _ _ _ _ _ _ _ _ _ _]
                frame -1, Default {
                }
                frame 0 {
                  n56 = call <vilib>:"sit CONVERT DBL.vi"("Last Row"=w206, "Raw Data"=w207) -> ("Output"=→"Bowthruster Battery":dbl)  [unwired: 9 in]
                }
                frame 1 {
                  n57 = call <vilib>:"sit CONVERT DBL.vi"("Last Row"=w209, "Raw Data"=w210) -> ("Output"=→"CSE1 pitch [rad]":dbl)  [unwired: 9 in]
                }
                frame 2 {
                  n58 = call <vilib>:"sit CONVERT DBL.vi"("Last Row"=w212, "Raw Data"=w213) -> ("Output"=→"CSE1 roll [rad]":dbl)  [unwired: 9 in]
                }
                frame 3 {
                  n59 = call <vilib>:"sit CONVERT DBL.vi"("Last Row"=w215, "Raw Data"=w216) -> ("Output"=→"CSE1 x-position [m]":dbl)  [unwired: 9 in]
                }
                frame 4 {
                  n60 = call <vilib>:"sit CONVERT DBL.vi"("Last Row"=w218, "Raw Data"=w219) -> ("Output"=→"CSE1 y-position [m]":dbl)  [unwired: 9 in]
                }
                frame 5 {
                  n61 = call <vilib>:"sit CONVERT DBL.vi"("Last Row"=w221, "Raw Data"=w222) -> ("Output"=→"CSE1 yaw [rad]":dbl)  [unwired: 9 in]
                }
                frame 6 {
                  n62 = call <vilib>:"sit CONVERT DBL.vi"("Last Row"=w224, "Raw Data"=w225) -> ("Output"=→"CSE1 z-position [m]":dbl)  [unwired: 9 in]
                }
                frame 7 {
                  n63 = call <vilib>:"sit CONVERT WaveformChart.vi"("Timestamps"=w227, "Last Row"=w228, "Raw Data"=w229) -> ("Output"=w226:waveform(dbl)[][])  [unwired: 8 in]
                  n64 = for {
                    tunnel: w226 -> [w230] mode=indexing
                    "DP Error E" <- w230
                  }
                }
                frame 8 {
                  n65 = call <vilib>:"sit CONVERT WaveformChart.vi"("Timestamps"=w232, "Last Row"=w233, "Raw Data"=w234) -> ("Output"=w231:waveform(dbl)[][])  [unwired: 8 in]
                  n66 = for {
                    tunnel: w231 -> [w235] mode=indexing
                    "DP Error N" <- w235
                  }
                }
                frame 9 {
                  n67 = call <vilib>:"sit CONVERT WaveformChart.vi"("Timestamps"=w237, "Last Row"=w238, "Raw Data"=w239) -> ("Output"=w236:waveform(dbl)[][])  [unwired: 8 in]
                  n68 = for {
                    tunnel: w236 -> [w240] mode=indexing
                    "DP Error Psi" <- w240
                  }
                }
                frame 10 {
                  n69 = call <vilib>:"sit CONVERT DBL.vi"("Last Row"=w242, "Raw Data"=w243) -> ("Output"=→"DP eta E":dbl)  [unwired: 9 in]
                }
                frame 11 {
                  n70 = call <vilib>:"sit CONVERT DBL.vi"("Last Row"=w245, "Raw Data"=w246) -> ("Output"=→"DP eta N":dbl)  [unwired: 9 in]
                }
                frame 12 {
                  n71 = call <vilib>:"sit CONVERT DBL.vi"("Last Row"=w248, "Raw Data"=w249) -> ("Output"=→"DP eta Psi deg":dbl)  [unwired: 9 in]
                }
                frame 13 {
                  n72 = call <vilib>:"sit CONVERT DBL.vi"("Last Row"=w251, "Raw Data"=w252) -> ("Output"=→"DP eta_d E":dbl)  [unwired: 9 in]
                }
                frame 14 {
                  n73 = call <vilib>:"sit CONVERT DBL.vi"("Last Row"=w254, "Raw Data"=w255) -> ("Output"=→"DP eta_d N":dbl)  [unwired: 9 in]
                }
                frame 15 {
                  n74 = call <vilib>:"sit CONVERT DBL.vi"("Last Row"=w257, "Raw Data"=w258) -> ("Output"=→"DP eta_d Psi deg":dbl)  [unwired: 9 in]
                }
                frame 16 {
                  n75 = call <vilib>:"sit CONVERT WaveformChart.vi"("Timestamps"=w260, "Last Row"=w261, "Raw Data"=w262) -> ("Output"=w259:waveform(dbl)[][])  [unwired: 8 in]
                  n76 = for {
                    tunnel: w259 -> [w263] mode=indexing
                    "DP tau surge" <- w263
                  }
                }
                frame 17 {
                  n77 = call <vilib>:"sit CONVERT WaveformChart.vi"("Timestamps"=w265, "Last Row"=w266, "Raw Data"=w267) -> ("Output"=w264:waveform(dbl)[][])  [unwired: 8 in]
                  n78 = for {
                    tunnel: w264 -> [w268] mode=indexing
                    "DP tau sway" <- w268
                  }
                }
                frame 18 {
                  n79 = call <vilib>:"sit CONVERT WaveformChart.vi"("Timestamps"=w270, "Last Row"=w271, "Raw Data"=w272) -> ("Output"=w269:waveform(dbl)[][])  [unwired: 8 in]
                  n80 = for {
                    tunnel: w269 -> [w273] mode=indexing
                    "DP tau yaw" <- w273
                  }
                }
                frame 19 {
                  n81 = call <vilib>:"sit CONVERT WaveformChart.vi"("Timestamps"=w275, "Last Row"=w276, "Raw Data"=w277) -> ("Output"=w274:waveform(dbl)[][])  [unwired: 8 in]
                  n82 = for {
                    tunnel: w274 -> [w278] mode=indexing
                    "DP u_1" <- w278
                  }
                }
                frame 20 {
                  n83 = call <vilib>:"sit CONVERT WaveformChart.vi"("Timestamps"=w280, "Last Row"=w281, "Raw Data"=w282) -> ("Output"=w279:waveform(dbl)[][])  [unwired: 8 in]
                  n84 = for {
                    tunnel: w279 -> [w283] mode=indexing
                    "DP u_2" <- w283
                  }
                }
                frame 21 {
                  n85 = call <vilib>:"sit CONVERT WaveformChart.vi"("Timestamps"=w285, "Last Row"=w286, "Raw Data"=w287) -> ("Output"=w284:waveform(dbl)[][])  [unwired: 8 in]
                  n86 = for {
                    tunnel: w284 -> [w288] mode=indexing
                    "DP u_3" <- w288
                  }
                }
                frame 22 {
                  n87 = call <vilib>:"sit CONVERT WaveformChart.vi"("Timestamps"=w290, "Last Row"=w291, "Raw Data"=w292) -> ("Output"=w289:waveform(dbl)[][])  [unwired: 8 in]
                  n88 = for {
                    tunnel: w289 -> [w293] mode=indexing
                    "DP u_4" <- w293
                  }
                }
                frame 23 {
                  n89 = call <vilib>:"sit CONVERT WaveformChart.vi"("Timestamps"=w295, "Last Row"=w296, "Raw Data"=w297) -> ("Output"=w294:waveform(dbl)[][])  [unwired: 8 in]
                  n90 = for {
                    tunnel: w294 -> [w298] mode=indexing
                    "DP u_5" <- w298
                  }
                }
                frame 24 {
                  n91 = call <vilib>:"sit CONVERT DBL.vi"("Last Row"=w300, "Raw Data"=w301) -> ("Output"=→"Direction Port VSP":dbl)  [unwired: 9 in]
                }
                frame 25 {
                  n92 = call <vilib>:"sit CONVERT DBL.vi"("Last Row"=w303, "Raw Data"=w304) -> ("Output"=→"Direction Starboard VSP":dbl)  [unwired: 9 in]
                }
                frame 26 {
                  n93 = call <vilib>:"sit CONVERT DBL.vi"("Last Row"=w306, "Raw Data"=w307) -> ("Output"=→"Iceberg pitch":dbl)  [unwired: 9 in]
                }
                frame 27 {
                  n94 = call <vilib>:"sit CONVERT DBL.vi"("Last Row"=w309, "Raw Data"=w310) -> ("Output"=→"Iceberg roll":dbl)  [unwired: 9 in]
                }
                frame 28 {
                  n95 = call <vilib>:"sit CONVERT DBL.vi"("Last Row"=w312, "Raw Data"=w313) -> ("Output"=→"Iceberg x-position":dbl)  [unwired: 9 in]
                }
                frame 29 {
                  n96 = call <vilib>:"sit CONVERT DBL.vi"("Last Row"=w315, "Raw Data"=w316) -> ("Output"=→"Iceberg y-position":dbl)  [unwired: 9 in]
                }
                frame 30 {
                  n97 = call <vilib>:"sit CONVERT DBL.vi"("Last Row"=w318, "Raw Data"=w319) -> ("Output"=→"Iceberg yaw":dbl)  [unwired: 9 in]
                }
                frame 31 {
                  n98 = call <vilib>:"sit CONVERT DBL.vi"("Last Row"=w321, "Raw Data"=w322) -> ("Output"=→"Iceberg z-position":dbl)  [unwired: 9 in]
                }
                frame 32 {
                  n99 = call <vilib>:"sit CONVERT DBL.vi"("Last Row"=w324, "Raw Data"=w325) -> ("Output"=→"LS  eta_surge_hil":dbl)  [unwired: 9 in]
                }
                frame 33 {
                  n100 = call <vilib>:"sit CONVERT DBL.vi"("Last Row"=w327, "Raw Data"=w328) -> ("Output"=→"LS eta_sway_hil":dbl)  [unwired: 9 in]
                }
                frame 34 {
                  n101 = call <vilib>:"sit CONVERT DBL.vi"("Last Row"=w330, "Raw Data"=w331) -> ("Output"=→"LS eta_yaw_hil":dbl)  [unwired: 9 in]
                }
                frame 35 {
                  n102 = call <vilib>:"sit CONVERT DBL.vi"("Last Row"=w333, "Raw Data"=w334) -> ("Output"=→"LS etadot_surge_hil":dbl)  [unwired: 9 in]
                }
                frame 36 {
                  n103 = call <vilib>:"sit CONVERT DBL.vi"("Last Row"=w336, "Raw Data"=w337) -> ("Output"=→"LS etadot_sway_hil":dbl)  [unwired: 9 in]
                }
                frame 37 {
                  n104 = call <vilib>:"sit CONVERT DBL.vi"("Last Row"=w339, "Raw Data"=w340) -> ("Output"=→"LS etadot_yaw_hil":dbl)  [unwired: 9 in]
                }
                frame 38 {
                  n105 = call <vilib>:"sit CONVERT DBL.vi"("Last Row"=w342, "Raw Data"=w343) -> ("Output"=→"LS nu_surge_hil":dbl)  [unwired: 9 in]
                }
                frame 39 {
                  n106 = call <vilib>:"sit CONVERT DBL.vi"("Last Row"=w345, "Raw Data"=w346) -> ("Output"=→"LS nu_sway_hil":dbl)  [unwired: 9 in]
                }
                frame 40 {
                  n107 = call <vilib>:"sit CONVERT DBL.vi"("Last Row"=w348, "Raw Data"=w349) -> ("Output"=→"LS nu_yaw_hil":dbl)  [unwired: 9 in]
                }
                frame 41 {
                  n108 = call <vilib>:"sit CONVERT DBL.vi"("Last Row"=w351, "Raw Data"=w352) -> ("Output"=→"Magnitude Pitch Port VSP":dbl)  [unwired: 9 in]
                }
                frame 42 {
                  n109 = call <vilib>:"sit CONVERT DBL.vi"("Last Row"=w354, "Raw Data"=w355) -> ("Output"=→"Magnitude Pitch Starboard VSP":dbl)  [unwired: 9 in]
                }
                frame 43 {
                  n110 = call <vilib>:"sit CONVERT DBL.vi"("Last Row"=w357, "Raw Data"=w358) -> ("Output"=→"Main Battery":dbl)  [unwired: 9 in]
                }
                frame 44 {
                  n111 = call <vilib>:"sit CONVERT DBL.vi"("Last Row"=w360, "Raw Data"=w361) -> ("Output"=→"Navigation eta surge":dbl)  [unwired: 9 in]
                }
                frame 45 {
                  n112 = call <vilib>:"sit CONVERT DBL.vi"("Last Row"=w363, "Raw Data"=w364) -> ("Output"=→"Navigation eta sway":dbl)  [unwired: 9 in]
                }
                frame 46 {
                  n113 = call <vilib>:"sit CONVERT DBL.vi"("Last Row"=w366, "Raw Data"=w367) -> ("Output"=→"Navigation eta yaw":dbl)  [unwired: 9 in]
                }
                frame 47 {
                  n114 = call <vilib>:"sit CONVERT DBL.vi"("Last Row"=w369, "Raw Data"=w370) -> ("Output"=→"Plant u1":dbl)  [unwired: 9 in]
                }
                frame 48 {
                  n115 = call <vilib>:"sit CONVERT DBL.vi"("Last Row"=w372, "Raw Data"=w373) -> ("Output"=→"Plant u2":dbl)  [unwired: 9 in]
                }
                frame 49 {
                  n116 = call <vilib>:"sit CONVERT DBL.vi"("Last Row"=w375, "Raw Data"=w376) -> ("Output"=→"Plant u3":dbl)  [unwired: 9 in]
                }
                frame 50 {
                  n117 = call <vilib>:"sit CONVERT DBL.vi"("Last Row"=w378, "Raw Data"=w379) -> ("Output"=→"Plant u4":dbl)  [unwired: 9 in]
                }
                frame 51 {
                  n118 = call <vilib>:"sit CONVERT DBL.vi"("Last Row"=w381, "Raw Data"=w382) -> ("Output"=→"Plant u5":dbl)  [unwired: 9 in]
                }
                frame 52 {
                  n119 = call <vilib>:"sit CONVERT DBL.vi"("Last Row"=w384, "Raw Data"=w385) -> ("Output"=→"QS pitch [rad]":dbl)  [unwired: 9 in]
                }
                frame 53 {
                  n120 = call <vilib>:"sit CONVERT DBL.vi"("Last Row"=w387, "Raw Data"=w388) -> ("Output"=→"QS roll [rad]":dbl)  [unwired: 9 in]
                }
                frame 54 {
                  n121 = call <vilib>:"sit CONVERT DBL.vi"("Last Row"=w390, "Raw Data"=w391) -> ("Output"=→"QS x-position [m]":dbl)  [unwired: 9 in]
                }
                frame 55 {
                  n122 = call <vilib>:"sit CONVERT DBL.vi"("Last Row"=w393, "Raw Data"=w394) -> ("Output"=→"QS y-position [m]":dbl)  [unwired: 9 in]
                }
                frame 56 {
                  n123 = call <vilib>:"sit CONVERT DBL.vi"("Last Row"=w396, "Raw Data"=w397) -> ("Output"=→"QS yaw [rad]":dbl)  [unwired: 9 in]
                }
                frame 57 {
                  n124 = call <vilib>:"sit CONVERT DBL.vi"("Last Row"=w399, "Raw Data"=w400) -> ("Output"=→"QS z-position [m]":dbl)  [unwired: 9 in]
                }
                frame 58 {
                  n125 = call <vilib>:"sit CONVERT DBL.vi"("Last Row"=w402, "Raw Data"=w403) -> ("Output"=→"QTM In1":dbl)  [unwired: 9 in]
                }
                frame 59 {
                  n126 = call <vilib>:"sit CONVERT DBL.vi"("Last Row"=w405, "Raw Data"=w406) -> ("Output"=→"QTM In2":dbl)  [unwired: 9 in]
                }
                frame 60 {
                  n127 = call <vilib>:"sit CONVERT DBL.vi"("Last Row"=w408, "Raw Data"=w409) -> ("Output"=→"QTM In3":dbl)  [unwired: 9 in]
                }
                frame 61 {
                  n128 = call <vilib>:"sit CONVERT DBL.vi"("Last Row"=w411, "Raw Data"=w412) -> ("Output"=→"QTM In4":dbl)  [unwired: 9 in]
                }
                frame 62 {
                  n129 = call <vilib>:"sit CONVERT DBL.vi"("Last Row"=w414, "Raw Data"=w415) -> ("Output"=→"QTM In5":dbl)  [unwired: 9 in]
                }
                frame 63 {
                  n130 = call <vilib>:"sit CONVERT DBL.vi"("Last Row"=w417, "Raw Data"=w418) -> ("Output"=→"QTM In6":dbl)  [unwired: 9 in]
                }
                frame 64 {
                  n131 = call <vilib>:"sit CONVERT DBL.vi"("Last Row"=w420, "Raw Data"=w421) -> ("Output"=→"QTM In7":dbl)  [unwired: 9 in]
                }
                frame 65 {
                  n132 = call <vilib>:"sit CONVERT DBL.vi"("Last Row"=w423, "Raw Data"=w424) -> ("Output"=→"QTM In8":dbl)  [unwired: 9 in]
                }
                frame 66 {
                  n133 = call <vilib>:"sit CONVERT DBL.vi"("Last Row"=w426, "Raw Data"=w427) -> ("Output"=→"QTM In9":dbl)  [unwired: 9 in]
                }
                frame 67 {
                  n134 = call <vilib>:"sit CONVERT DBL.vi"("Last Row"=w429, "Raw Data"=w430) -> ("Output"=→"Servo Battery":dbl)  [unwired: 9 in]
                }
                frame 68 {
                  n135 = call <vilib>:"sit CONVERT DBL.vi"("Last Row"=w432, "Raw Data"=w433) -> ("Output"=→"Slide BT green":dbl)  [unwired: 9 in]
                }
                frame 69 {
                  n136 = call <vilib>:"sit CONVERT DBL.vi"("Last Row"=w435, "Raw Data"=w436) -> ("Output"=→"Slide BT red":dbl)  [unwired: 9 in]
                }
              }
            }
          }
        }
        n137 = call <vilib>:"sit Check to Stop Client.vi"("error in (no error)"=w182) -> ("error out"=w183:errorcluster, "Stop?"=w181:bool)  [unwired: 2 in, 7 out]
        n138 = Wait (ms)(milliseconds to wait=u32 50) -> ()  [unwired: 1 out]
      }
      n139 = local write "SIT_Meta_Info"(w88) -> ()
      n140 = call <vilib>:"sit Merge SIT Client Errors.vi"("Bottom Loop Error"=w84, "Top Loop Error"=w82) -> ("Resulting Error"=w83:errorcluster)  [unwired: 9 out]
    }
    frame Error {
      # "User canceled target selection (or an error occurred on Init)...don't run the client"
      n141 = local write "SIT_Meta_Info"(w437) -> ()
    }
  }
  n142 = Current VI's Path() -> (path=w47:path)
  n143 = Current VI's Path() -> (path=w20:path)
  n144 = Current VI's Path() -> (path=w25:path)
  n145 = Strip Path(path=w47) -> (stripped path=w46:path)  [unwired: 1 out]
  n146 = Strip Path(path=w20) -> (stripped path=w19:path)  [unwired: 1 out]
  n147 = Strip Path(path=w25) -> (stripped path=w24:path)  [unwired: 1 out]
  n148 = Build Path(base path=w46, name or relative path="model\\3D\\3dsboat55.wrl" ("Name")) -> (appended path=w43:path)
  n149 = call <vilib>:"Create Box.vi"("Color"=T11 {"Red"=0.0, "Green"=0.0, "Blue"=1.0, "Alpha"=1.0}, "Length Z"=sgl 6.5 ("Red"), "Length Y"=sgl 0.001 ("Red"), "Length X"=sgl 20.0 ("Red")) -> ("New Box Refnum"=w50:refnum<vi>)  [unwired: 6 in, 1 out]
  n150 = call <vilib>:"Create Object.vi"("Name"="Sea") -> ("Scene:New Object"=w51:refnum<vi>)  [unwired: 9 in, 1 out]
  n151 = Build Path(base path=w19, name or relative path="model\\3D\\iceberg2.wrl" ("Name")) -> (appended path=w16:path)
  n152 = Build Path(base path=w24, name or relative path="model\\3D\\target2.wrl" ("Name")) -> (appended path=w22:path)
  n153 = call <vilib>:"Load VRML File.vi"("Path"=w43) -> ("Scene:Read Scene File"=w42:refnum<vi>)  [unwired: 9 in, 1 out]
  n154 = call <vilib>:"Create Object.vi"("Name"="Ship") -> ("Scene:New Object"=w44:refnum<vi>)  [unwired: 9 in, 1 out]
  n155 = call <vilib>:"Load VRML File.vi"("Path"=w16) -> ("Scene:Read Scene File"=w15:refnum<vi>)  [unwired: 9 in, 1 out]
  n156 = call <vilib>:"Create Object.vi"("Name"="Iceberg") -> ("Scene:New Object"=w17:refnum<vi>)  [unwired: 9 in, 1 out]
  n157 = call <vilib>:"Load VRML File.vi"("Path"=w22) -> ("Scene:Read Scene File"=w21:refnum<vi>)  [unwired: 9 in, 1 out]
  n158 = invoke on="Invoke Node" class="SceneObject" method="Set Drawable"(reference=w51, "Drawable"=w50) -> (reference out=w39:refnum<vi>)  [unwired: 2 in, 3 out]
  n159 = while "Input Signal handeling from PS3 device" {
    tunnel: w59 -> [w498]
    tunnel: w58 -> [w497]
    tunnel: [w462] -> w54
    tunnel: [w463] -> w53
    stop <- w458 stop-if-true
    w464 = 0.1  # Step length
    w476 = 0.1  # Step length
    # "PS3 Signal updates every\n100 millisecond (10 Hz)\nmodify by editing number in\nblue box"
    # "Threshold preventing chattering"
    n160 = call-poly <vilib>:"Acquire Input Data.vi"("device ID"=w498, "error in (no error)"=w497) -> ("device ID"=w462:refnum<k1>, "axis info"=w494:T17, "button info"=w496:T18, "direction info"=w495:T19, "error out"=w463:errorcluster)  [unwired: 13 in]
    n161 = Unbundle By Name "Button info"(w496) -> ("button 1"=→"Square Button":bool, "button 2"=→"X Button":bool, "button 3"=→"Circle Button":bool, "button 4"=→"Triangle Button":bool, "button 7"=w456:bool, "button 8"=w457:bool, "button 9"=w480:bool, "button 10"=w468:bool, "button 11"=w479:bool, "button 12"=w467:bool)  [unwired: 2 out]
    "R2 Button" <- w456
    "L2 Button" <- w457
    "Direction Left" <- w480
    "Direction Down" <- w468
    "Direction Right" <- w479
    "Direction Up" <- w467
    n162 = Unbundle By Name "Direction info"(w495) -> ()  [unwired: 4 out]
    n163 = Unbundle By Name "Axis info"(w494) -> ("X axis"=w444:i32, "Y axis"=w493:i32, "Z axis"=w442:i32, "U axis"=w492:i32)  [unwired: 4 out]
    n164 = Negate(x=w492) -> (-x=w441:i32)
    n165 = Negate(x=w493) -> (-x=w443:i32)
    n166 = property on="Left Stick X" class="Slide (strict)"("Val(Sgnl)"=w444) -> ()  [unwired: 2 in, 2 out]
    n167 = property on="Right Stick X" class="Slide (strict)"("Val(Sgnl)"=w442) -> ()  [unwired: 2 in, 2 out]
    n168 = property on="Right Stick Y" class="Slide (strict)"("Val(Sgnl)"=w441) -> ()  [unwired: 2 in, 2 out]
    n169 = property on="Left Stick Y" class="Slide (strict)"("Val(Sgnl)"=w443) -> ()  [unwired: 2 in, 2 out]
    n170 = Boolean To (0,1)(Boolean=w456) -> (0, 1=w455:i16)
    n171 = Boolean To (0,1)(Boolean=w457) -> (0, 1=w452:i16)
    n172 = Negate(x=w455) -> (-x=w451:i16)
    n173 = Square(x=w442) -> (x^2=w449:i32)
    n174 = Square(x=w441) -> (x^2=w450:i32)
    n175 = Square(x=w444) -> (x^2=w447:i32)
    n176 = Square(x=w443) -> (x^2=w448:i32)
    n177 = property on="R2" class="DigNum (strict)"("Val(Sgnl)"=w451) -> ()  [unwired: 2 in, 2 out]
    n178 = property on="L2" class="DigNum (strict)"("Val(Sgnl)"=w452) -> ()  [unwired: 2 in, 2 out]
    n179 = feedback #1() -> (w485:bool)  [unwired: 1 in]
    n180 = feedback-in #1(w480) -> ()
    n181 = feedback #2() -> (w487:bool)  [unwired: 1 in]
    n182 = feedback-in #2(w479) -> ()
    n183 = feedback #3() -> (w473:bool)  [unwired: 1 in]
    n184 = feedback-in #3(w468) -> ()
    n185 = feedback #4() -> (w475:bool)  [unwired: 1 in]
    n186 = feedback-in #4(w467) -> ()
    n187 = Add(x=w447, y=w448) -> (x+y=w445:i32)
    n188 = Add(x=w449, y=w450) -> (x+y=w446:i32)
    n189 = Greater?(x=w480, y=w485) -> (0:w484:bool)
    n190 = Greater?(x=w479, y=w487) -> (0:w486:bool)
    n191 = Greater?(x=w468, y=w473) -> (0:w472:bool)
    n192 = Greater?(x=w467, y=w475) -> (0:w474:bool)
    n193 = Square Root(x=w445) -> (sqrt(x)=w440:dbl)
    n194 = Square Root(x=w446) -> (sqrt(x)=w439:dbl)
    n195 = call <vilib>:"Increment PtByPt.vi"("activate"=w484) -> ("counter"=w483:u32)  [unwired: 1 in, 1 out]
    n196 = call <vilib>:"Increment PtByPt.vi"("activate"=w486) -> ("counter"=w478:u32)  [unwired: 1 in, 1 out]
    n197 = call <vilib>:"Increment PtByPt.vi"("activate"=w472) -> ("counter"=w471:u32)  [unwired: 1 in, 1 out]
    n198 = call <vilib>:"Increment PtByPt.vi"("activate"=w474) -> ("counter"=w465:u32)  [unwired: 1 in, 1 out]
    n199 = To Double Precision Float(number=w483) -> (double precision float=w482:dbl)
    n200 = To Double Precision Float(number=w471) -> (double precision float=w470:dbl)
    n201 = call "Out of Range"("Operand 1"=w440) -> ("Result"=→"Left Joystick":dynamicdata)  [unwired: 9 in, 1 out]
    n202 = call "Out of Range"("Operand 1"=w439) -> ("Result"=→"Right Joystick":dynamicdata)  [unwired: 9 in, 1 out]
    n203 = Negate(x=w482) -> (-x=w481:dbl)
    n204 = Negate(x=w470) -> (-x=w466:dbl)
    n205 = Add(x=w481, y=w478) -> (x+y=w477:dbl)
    n206 = Add(x=w466, y=w465) -> (x+y=w469:dbl)
    n207 = Multiply(x=w477, y=w476) -> (x*y=w454:dbl)
    n208 = Multiply(x=w469, y=w464) -> (x*y=w453:dbl)
    n209 = property on="BT Power Limiter" class="Slide (strict)"("Val(Sgnl)"=w454) -> ()  [unwired: 2 in, 2 out]
    n210 = property on="VSP Speed" class="Slide (strict)"("Val(Sgnl)"=w453) -> ()  [unwired: 2 in, 2 out]
    n211 = property on="SIT_stopVI" class="Bool (strict)"() -> ("Value"=w458:bool)  [unwired: 2 in, 2 out]
    n212 = Wait (ms)(milliseconds to wait=u32 100) -> ()  [unwired: 1 out]
  }
  n213 = invoke on="Invoke Node" class="SceneObject" method="Object.Add Object"(reference=w44, "Child"=w42) -> (reference out=w38:refnum<vi>, "Child"=w37:refnum<vi>)  [unwired: 2 in, 2 out]
  n214 = invoke on="Invoke Node" class="SceneObject" method="Object.Add Object"(reference=w17, "Child"=w15) -> (reference out=w9:refnum<vi>, "Child"=w13:refnum<vi>)  [unwired: 2 in, 2 out]
  n215 = call <vilib>:"Create Object.vi"("Name"="DP waypoint") -> ("Scene:New Object"=w36:refnum<vi>)  [unwired: 9 in, 1 out]
  n216 = invoke on="3D Picture" class="SceneGraphDisp (strict)" method="Setup Camera"("Camera Position"=cluster{"X":sgl, "Y":sgl, "Z":sgl} {"X"=-15.0, "Y"=11.0, "Z"=0.0}, "Target"=cluster{"X":sgl, "Y":sgl, "Z":sgl} {"X"=0.0, "Y"=0.0, "Z"=0.0} ("Camera Position"), "Up Direction"=cluster{"X":sgl, "Y":sgl, "Z":sgl} {"X"=1.0, "Y"=0.0, "Z"=0.0} ("Camera Position")) -> ()  [unwired: 3 in, 6 out]
  n217 = property on="SIT_Run" class="Bool (strict)"() -> ("Value"=w1:bool)  [unwired: 2 in, 2 out]
  n218 = call <vilib>:"Set Scale.vi"("Scale"=cluster{"X":sgl, "Y":sgl, "Z":sgl} {"X"=0.001, "Y"=0.001, "Z"=0.001} ("Initial Position"), "Scene Object"=w37) -> ("Scaled Object"=w8:refnum<vi>)  [unwired: 8 in, 1 out]
  n219 = call <vilib>:"Set Scale.vi"("Scale"=cluster{"X":sgl, "Y":sgl, "Z":sgl} {"X"=0.001, "Y"=0.001, "Z"=0.001} ("Initial Position"), "Scene Object"=w13) -> ("Scaled Object"=w6:refnum<vi>)  [unwired: 8 in, 1 out]
  n220 = invoke on="Invoke Node" class="SceneObject" method="Object.Add Object"(reference=w36, "Child"=w21) -> (reference out=w31:refnum<vi>, "Child"=w7:refnum<vi>)  [unwired: 2 in, 2 out]
  n221 = invoke on="Invoke Node" class="SceneObject" method="Object.Add Object"(reference=w39, "Child"=w38) -> (reference out=w34:refnum<vi>)  [unwired: 2 in, 3 out]
  n222 = case shown="True" w1 {
    frame False {
    }
    frame True {
      n223 = while {
        stop <- w500 stop-if-true
        # "Response charts DP"
        # "Response chart adds new point every\n100 milliseconds (10 Hz)\nmodify by editing blue box number"
        n224 = local read "DP eta_d N"() -> (w508:dbl)
        n225 = local read "DP eta N"() -> (w509:dbl)
        n226 = property on="DP eta Psi deg" class="DigNum (strict)"() -> ("Value"=w505:dbl)  [unwired: 2 in, 2 out]
        n227 = property on="DP eta_d Psi deg" class="DigNum (strict)"() -> ("Value"=w502:dbl)  [unwired: 2 in, 2 out]
        n228 = property on="DP eta E" class="DigNum (strict)"() -> ("Value"=w503:dbl)  [unwired: 2 in, 2 out]
        n229 = property on="DP eta_d E" class="DigNum (strict)"() -> ("Value"=w501:dbl)  [unwired: 2 in, 2 out]
        n230 = Bundle("Value"=w501, "Value"=w503) -> (→"DP Response E":cluster{"Value":dbl, "Value":dbl})  [unwired: 1 in]
        n231 = Bundle("Value"=w502, "Value"=w505) -> (→"DP Reponse Psi":cluster{"Value":dbl, "Value":dbl})  [unwired: 1 in]
        n232 = Bundle("DP eta_d N"=w508, "DP eta N"=w509) -> (→"DP Reponse N":cluster{"DP eta_d N":dbl, "DP eta N":dbl})  [unwired: 1 in]
        n233 = property on="SIT_Stop" class="Bool (strict)"() -> ("Value"=w500:bool)  [unwired: 2 in, 2 out]
        n234 = Wait (ms)(milliseconds to wait=u32 100) -> ()  [unwired: 1 out]
      }
    }
  }
  n235 = local write "SIT_stopVI"(w66) -> ()
  n236 = call <vilib>:"sit Clear Client.vi"("error in (no error)"=w72, "SIT Client Op Refs"=w68) -> ("error out"=w69:errorcluster)  [unwired: 9 out]
  n237 = call <vilib>:"sit Check to Stop Client.vi"("Reset Stop?"=TRUE ("Clear Item?"), "error in (no error)"=w69) -> ("error out"=w61:errorcluster)  [unwired: 1 in, 8 out]
  n238 = property on="3D Picture" class="SceneGraphDisp (strict)"("Background Color"=cluster{"X":sgl, "Y":sgl, "Z":sgl, "Z 2":sgl} {"X"=1.0, "Y"=1.0, "Z"=1.0, "Z 2"=1.0} ("Camera Position")) -> ()  [unwired: 2 in, 2 out]
  n239 = call <vilib>:"sit Check Run-Time System.vi"("error in"=w61) -> ("Run Time System?"=w60:bool)  [unwired: 10 out]
  n240 = Quit LabVIEW(quit? (T)=w60) -> ()
  n241 = invoke on="Invoke Node" class="SceneObject" method="Object.Add Object"(reference=w34, "Child"=w31) -> (reference out=w10:refnum<vi>)  [unwired: 2 in, 3 out]
  n242 = invoke on="Invoke Node" class="SceneObject" method="Object.Add Object"(reference=w10, "Child"=w9) -> (reference out=w11:refnum<vi>)  [unwired: 2 in, 3 out]
  n243 = call-poly <vilib>:"Close Input Device.vi"("error in (no error)"=w53, "device ID"=w54) -> ("error out"=w52:errorcluster)  [unwired: 8 in]
  n244 = while {
    tunnel: w11 -> [w544]
    tunnel: w8 -> [w554]
    tunnel: w7 -> [w552]
    tunnel: w6 -> [w516]
    stop <- w543 stop-if-true
    # "3D display updates every\n100 miliseconds (10 Hz)\nmodify by editing the\nblue box number"
    # "yaw -> rotate around \ny-axis of  model"
    # "xzy due to boat bottom to top direction is along y-axis"
    # "yaw -> rotate around \ny-axis of boat model"
    # "yaw -> rotate around \ny-axis of model"
    # "xzy due to boat bottom to top direction is along y-axis"
    n245 = property on="CSE1 x-position [m]" class="DigNum (strict)"() -> ("Value"=w540:dbl)  [unwired: 2 in, 2 out]
    n246 = property on="CSE1 z-position [m]" class="DigNum (strict)" props=["Value"]() -> ()  [unwired: 2 in, 3 out]
    n247 = property on="CSE1 y-position [m]" class="DigNum (strict)"() -> ("Value"=w537:dbl)  [unwired: 2 in, 2 out]
    n248 = Not(x="Show CSEI") -> (.not. x?=w533:bool)
    n249 = property on="Iceberg x-position" class="DigNum (strict)"() -> ("Value"=w524:dbl)  [unwired: 2 in, 2 out]
    n250 = property on="Iceberg z-position" class="DigNum (strict)" props=["Value"]() -> ()  [unwired: 2 in, 3 out]
    n251 = property on="Iceberg y-position" class="DigNum (strict)"() -> ("Value"=w521:dbl)  [unwired: 2 in, 2 out]
    n252 = Boolean To (0,1)(Boolean=w533) -> (0, 1=w536:i16)
    n253 = Multiply(x=w537, y=1) -> (x*y=w538:dbl)
    n254 = Not(x="Show Iceberg") -> (.not. x?=w518:bool)
    n255 = Multiply(x=w540, y=1) -> (x*y=w541:dbl)
    n256 = Multiply(x="DP eta_d_Psi [deg]", y=3.141592653589793) -> (x*y=w512:dbl)
    n257 = Boolean To (0,1)(Boolean=w518) -> (0, 1=w520:i16)
    n258 = Bundle("DP eta_d_N [m]"="DP eta_d_N [m]", "Red"=sgl 0.0, "DP eta_d_E [m]"="DP eta_d_E [m]") -> (w548:T20)  [unwired: 1 in]
    n259 = Multiply(x=w521, y=1) -> (x*y=w522:dbl)
    n260 = Multiply(x=w524, y=1) -> (x*y=w525:dbl)
    n261 = Multiply(x=w536, y=-1) -> (x*y=w532:i32)
    n262 = Divide(x=w512, y=180) -> (x/y=w510:dbl)
    "Ind eta_d_Psi [rad]" <- w510
    n263 = Bundle(w541, w532, w538) -> (w553:cluster{dbl, i32, dbl})  [unwired: 1 in]
    n264 = call <vilib>:"Set Translation.vi"("Translation"=w548, "Scene Object"=w552) -> ("Translated Object"=w547:refnum<vi>)  [unwired: 8 in, 1 out]
    n265 = Multiply(x=w520, y=-1) -> (x*y=w517:i32)
    n266 = Bundle(w525, w517, w522) -> (w527:cluster{dbl, i32, dbl})  [unwired: 1 in]
    n267 = Negate(x=w510) -> (-x=w545:dbl)
    n268 = property on="CSE1 pitch [rad]" class="DigNum (strict)" props=["Value"]() -> ()  [unwired: 2 in, 3 out]
    n269 = property on="CSE1 yaw [rad]" class="DigNum (strict)"() -> ("Value"=w556:dbl)  [unwired: 2 in, 2 out]
    n270 = property on="CSE1 roll [rad]" class="DigNum (strict)" props=["Value"]() -> ()  [unwired: 2 in, 3 out]
    n271 = call <vilib>:"Set Translation.vi"("Translation"=w553, "Scene Object"=w554) -> ("Translated Object"=w558:refnum<vi>)  [unwired: 8 in, 1 out]
    n272 = call <vilib>:"Set Rotation.vi"("Angle"=w545, "Axis"=cluster{"X":sgl, "Y":sgl, "Z":sgl} {"X"=0.0, "Y"=1.0, "Z"=0.0} ("Camera Position"), "Scene Object"=w547) -> ()  [unwired: 7 in, 2 out]
    n273 = property on="Iceberg pitch" class="DigNum (strict)" props=["Value"]() -> ()  [unwired: 2 in, 3 out]
    n274 = property on="Iceberg yaw" class="DigNum (strict)"() -> ("Value"=w529:dbl)  [unwired: 2 in, 2 out]
    n275 = property on="Iceberg roll" class="DigNum (strict)" props=["Value"]() -> ()  [unwired: 2 in, 3 out]
    n276 = Negate(x=w556) -> (-x=w555:dbl)
    n277 = call <vilib>:"Set Translation.vi"("Translation"=w527, "Scene Object"=w516) -> ("Translated Object"=w531:refnum<vi>)  [unwired: 8 in, 1 out]
    n278 = property on="SIT_stopVI" class="Bool (strict)"() -> ("Value"=w543:bool)  [unwired: 2 in, 2 out]
    n279 = Negate(x=w529) -> (-x=w528:dbl)
    n280 = Wait (ms)(milliseconds to wait=u32 100) -> ()  [unwired: 1 out]
    n281 = call <vilib>:"Set Rotation.vi"("Angle"=w555, "Axis"=cluster{"X":sgl, "Y":sgl, "Z":sgl} {"X"=0.0, "Y"=1.0, "Z"=0.0} ("Camera Position"), "Scene Object"=w558) -> ()  [unwired: 7 in, 2 out]
    n282 = call <vilib>:"Set Rotation.vi"("Angle"=w528, "Axis"=cluster{"X":sgl, "Y":sgl, "Z":sgl} {"X"=0.0, "Y"=1.0, "Z"=0.0} ("Camera Position"), "Scene Object"=w531) -> ()  [unwired: 7 in, 2 out]
    "3D Picture" <- w544
  }
  n283 = call <vilib>:"General Error Handler.vi"("error in (no error)"=w52) -> ()  [unwired: 10 in, 5 out]
